vi "Send Match idot to shot.vi"(6 "# Copies (0 = infinite repeat)":u32=1, 7 "Message Priority (Normal)":T2=enum."Normal", 8 "error in (no error)":errorcluster, 9 "Delay message, ms":i32, 10 "Idot match record":T1, 11 "Message Enqueuer":refnum<class "Message Enqueuer.lvclass">) -> (0 "error out":errorcluster, 3 "Message Enqueuer out":refnum<class "Message Enqueuer.lvclass">)   [LabVIEW 2015, in "Match idot to shot Msg.lvclass"]
doc: "This VI sends the message to an actor."
uses:
  Match idot to shot Msg.lvclass
  <vilib>/ActorFramework/Message Enqueuer/Message Enqueuer.lvclass
  <vilib>/ActorFramework/Message Enqueuer/Message Priority.ctl
  Cap Bank Server/Idot match record.ctl
  Match idot to shot Msg.lvclass/Match idot to shot Msg.ctl
  <vilib>/ActorFramework/Message Enqueuer/Message Enqueuer.lvclass/Message Enqueuer.ctl
  <vilib>/ActorFramework/Message Priority Queue/Priority Enqueue.vi
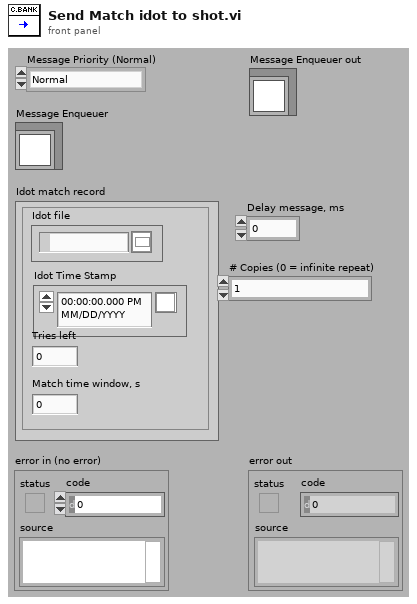
[diagram p1: front panel]
types:
  T1 = typedef "Idot match record.ctl" = cluster{"Idot file":path, "Idot Time Stamp":timestamp, "Tries left":i32, "Match time window, s":dbl}
  T2 = typedef "Actor Framework.lvlib/Message Enqueuer.lvclass/Message Priority.ctl" = enum16{"Low", "Normal", "High"}
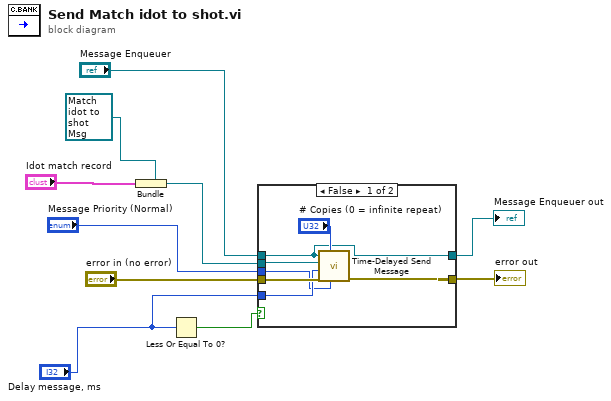
[diagram p0: block diagram]
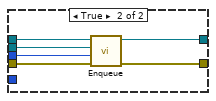
[diagram p2: hidden frame]
diagram:
  n1 = Bundle(cluster=refnum<class "Match idot to shot Msg.lvclass"> refnum ("Object"), "Idot match record") -> (w6:refnum<class "Match idot to shot Msg.lvclass">)
  n2 = Less Or Equal To 0?(x="Delay message, ms") -> (x <= 0?=w2:bool)
  n3 = case shown="False" w2 {
    tunnel: "Message Enqueuer" -> [w14 w23]
    tunnel: "error in (no error)" -> [w16 w22]
    tunnel: [w15 w21] -> w8
    tunnel: w6 -> [w13 w20]
    tunnel: "Message Priority (Normal)" -> [w11 w19]
    tunnel: [w14 w18] -> w4
    tunnel: "Delay message, ms" -> [w12 _]
    frame False {
      n4 = call <vilib>:"Time-Delayed Send Message.vi"("Message Priority (Normal)"=w11, "# Copies (0 = infinite repeat)"="# Copies (0 = infinite repeat)", "error in (no error)"=w16, "Milliseconds To Wait"=w12, "Message"=w13, "Message Enqueuer"=w14) -> ("error out"=w15:errorcluster)  [unwired: 4 in, 1 out]
    }
    frame True {
      n5 = call <vilib>:"Enqueue.vi"("error in (no error)"=w22, "Message Priority (Normal)"=w19, "Message"=w20, "Message Enqueuer in"=w23) -> ("error out"=w21:errorcluster, "Message Enqueuer out"=w18:refnum<class "Message Enqueuer.lvclass">)  [unwired: 6 in]
    }
  }
  "error out" <- w8
  "Message Enqueuer out" <- w4
